vi "ReadAndSaveData.vi"(0 "object in":refnum<class "CetoniPump.lvclass">, 2 "tdms file":refnum<k34>, 5 "error in (no error)":errorcluster) -> (14 "object out":refnum<class "CetoniPump.lvclass">, 19 "error out":errorcluster)   [LabVIEW 2023, in "CetoniPump.lvclass"]
uses:
  CetoniPump.lvclass
  CetoniPump.lvclass/CetoniPump.ctl
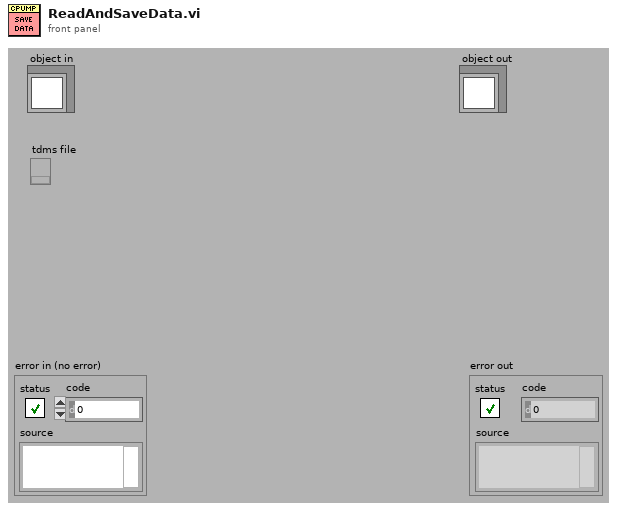
[diagram p1: front panel]
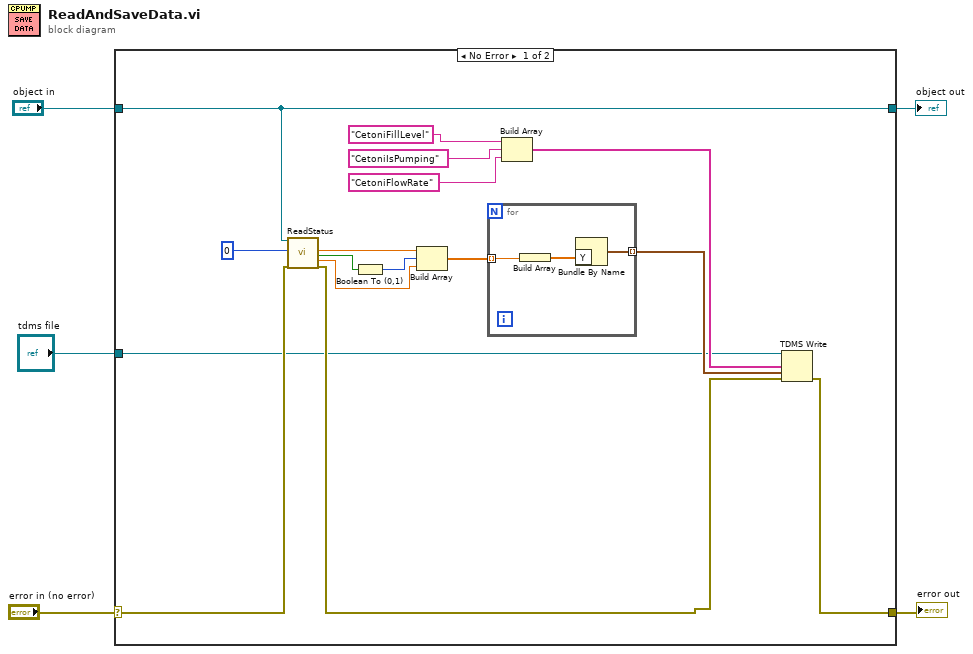
[diagram p0: block diagram]
diagram:
  n1 = case shown="No Error" "error in (no error)" {
    selector: "error in (no error)" -> [w19 w26]
    tunnel: [w7 w26] -> w4
    tunnel: [w21 w25] -> w2
    tunnel: "object in" -> [w21 w25]
    tunnel: "tdms file" -> [w6 _]
    frame No Error {
      n2 = call-dynamic "ReadStatus.vi"("object in"=w21, "index"=0, "error in (no error)"=w19) -> ("Fill Level"=w18:dbl, "Is pumping"=w17:bool, "Actual Flow Rate"=w15:dbl, "error out"=w8:errorcluster)  [unwired: 12 in, 1 out]
      n3 = Boolean To (0,1)(Boolean=w17) -> (0, 1=w16:i16)
      n4 = Build Array(w18, w16, w15) -> (w14:dbl[])
      n5 = for {
        tunnel: w14 -> [w24] mode=indexing
        tunnel: [w22] -> w9 mode=indexing
        n6 = Build Array(w24) -> (w23:dbl[])
        n7 = Bundle By Name("Y"=w23) -> (w22:waveform(dbl))  [unwired: 1 in]
      }
      n8 = Build Array("CetoniFillLevel", "CetoniIsPumping", "CetoniFlowRate") -> (w10:string[])
      n9 = TDMS Write(0:w6, 7:w10, 9:w9, 11:w8) -> (15:w7:errorcluster)  [unwired: 2 in, 3 out]
    }
    frame Error {
    }
  }
  "error out" <- w4
  "object out" <- w2
